vi "Control Panel (New).vi"(8 "error in (no error)":errorcluster, 11 "Lockin SR830 in":refnum<class "Lockin SR830.lvclass">) -> (0 "error out":errorcluster, 3 "Lockin SR830 out":refnum<class "Lockin SR830.lvclass">)   [LabVIEW 2017, in "Lockin SR830.lvclass"]
uses:
  Lockin SR830.lvclass
  Lockin SR830.lvclass/Lockin SR830.ctl
  sr830/SR830.lvlib
panel:
  in  "Read":bool
  in  "Read Dwell Time":dbl[unit] format="%^#_6g"
  out "Ref Freq":dbl[unit]
  out "R":dbl
  out "Y":dbl
  out "X":dbl
  out "Phase":dbl format="%#_13g"
  in  "autophase":bool
  out "External ref":bool=TRUE
  in  "External ref?":bool=TRUE
  in  "Read settings":bool
  in  "Copy actual to set":bool
  in  "Populate fields with member data":bool
  in  "endprgm":bool
  in  "set":bool
  out "sensdisp":T1(ring) caption="Sensitivity"
  out "tcdisp":T2(ring) caption="Time Const."
  in  "sens":T1(ring) caption="Sensitivity"
  in  "tc":T2(ring) caption="Time Const."
  # "Lock-in Detector Front Panel"
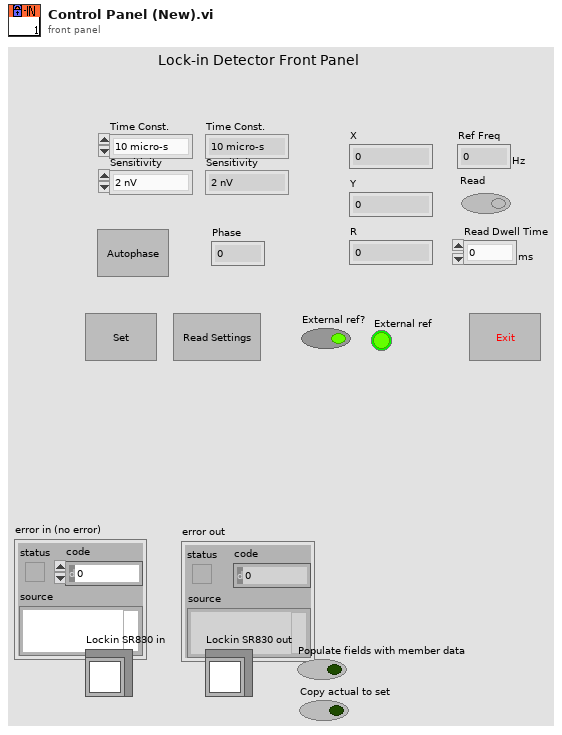
[diagram p1: front panel]
types:
  T1 = enum16{"2 nV", "5 nV", "10 nV", "20 nV", "50 nV", "100 nV", "200 nV", "500 nV", "1 microV", "2 microV", "5 microV", "10 microV", "20 microV", "50  microV", "100  microV", "200  microV", "500  microV", "1 mV", "2 mV", "5 mV", "10 mV", "20 mV", "50 mV", "100 mV", "200  mV", "500 mV", "1 V"}
  T2 = enum16{"10 micro-s", "30 micro-s", "100 micro-s", "300 micro-s", "1 ms", "3 ms", "10 ms", "30 ms", "100 ms", "300 ms", "1 s", "3 s", "10 s", "30 s", "100 s", "300 s", "1000 s", "30000 s", "10 ks", "30 ks"}
  T3 = typedef "Lockin SR830.lvclass/Sensitivity.ctl" = u16
  T4 = typedef "SR830.lvlib/Tau.ctl" = u16
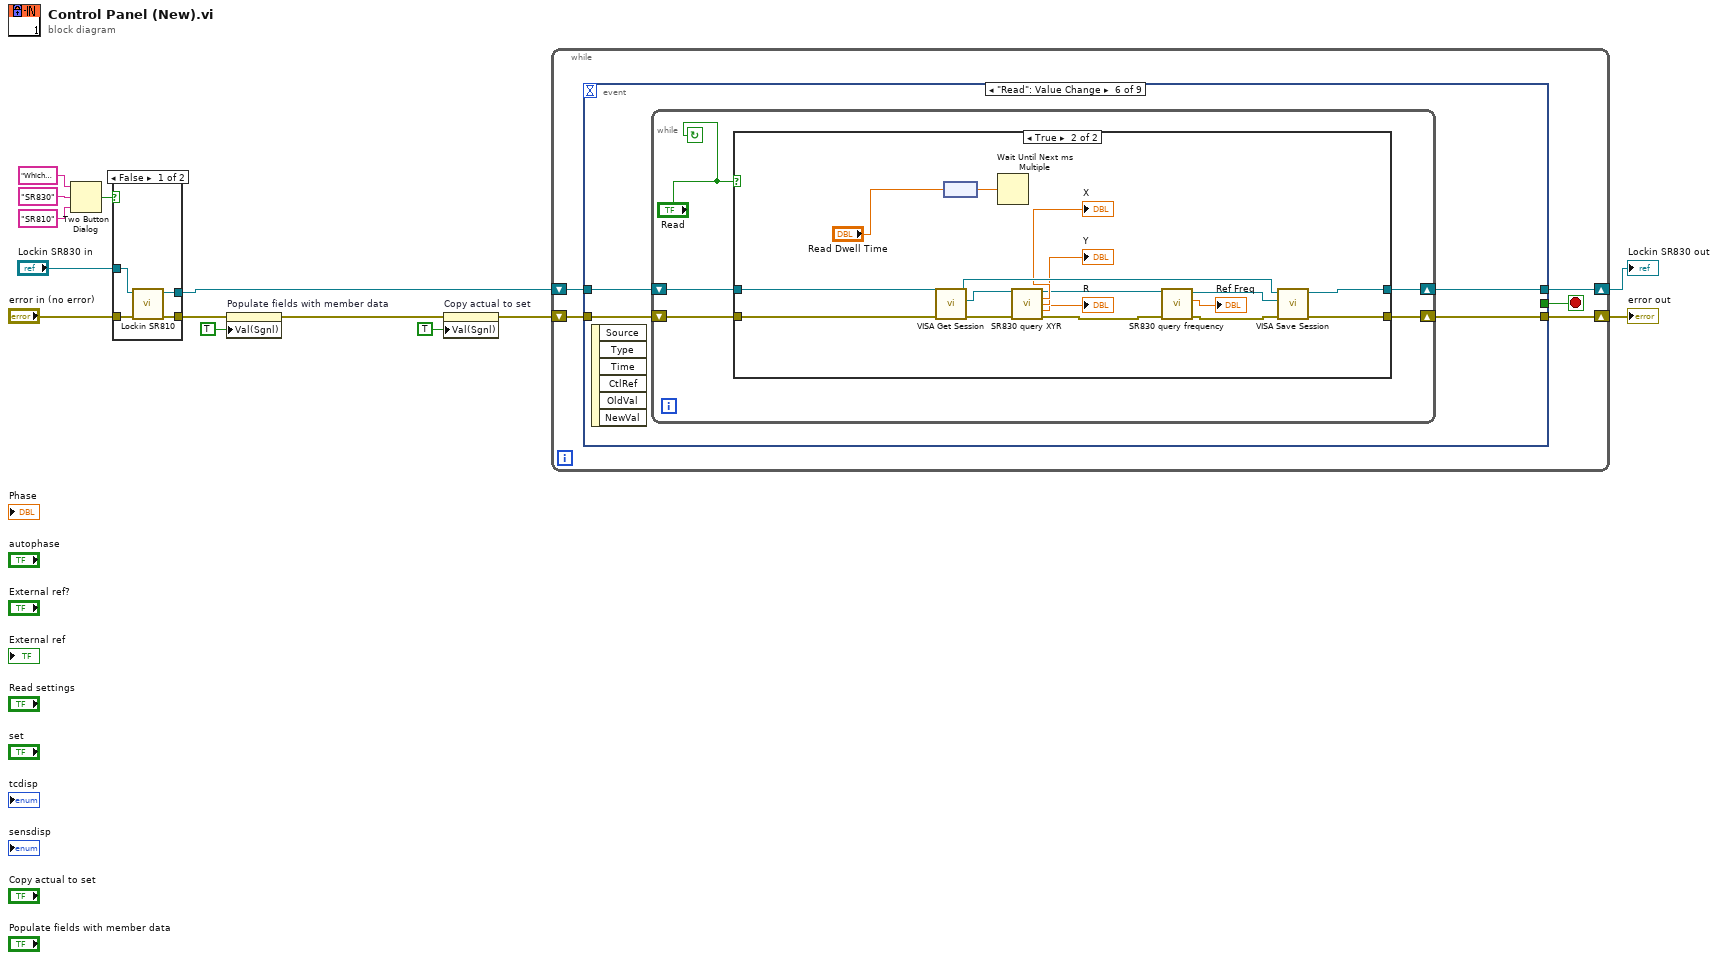
[diagram p0: block diagram]
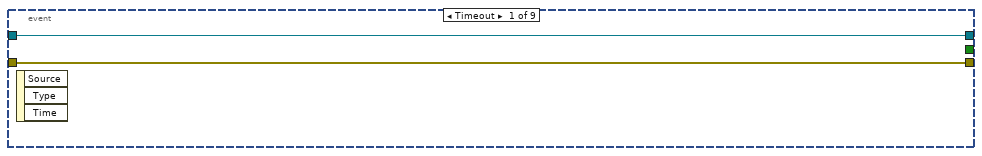
[diagram p2: hidden frame]
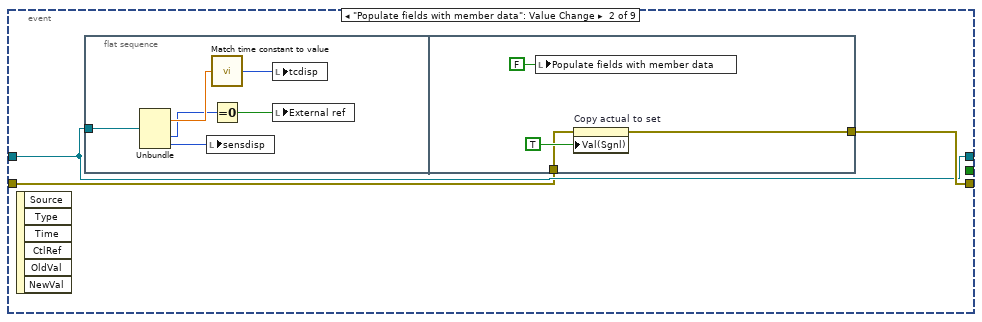
[diagram p3: hidden frame]
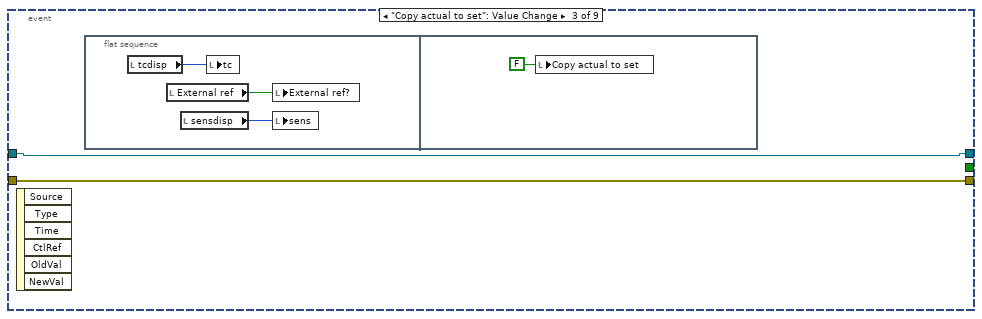
[diagram p4: hidden frame]
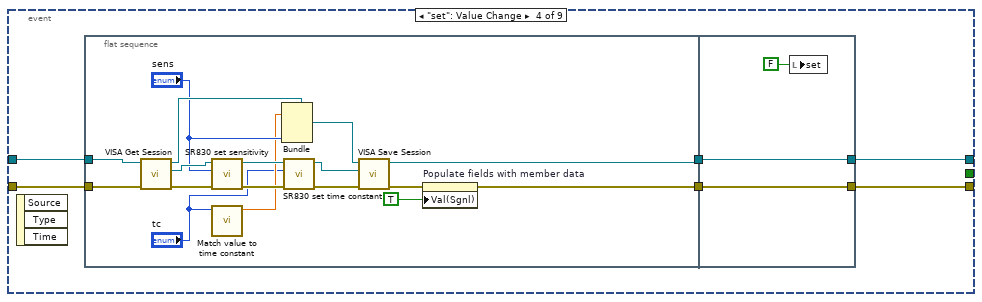
[diagram p5: hidden frame]
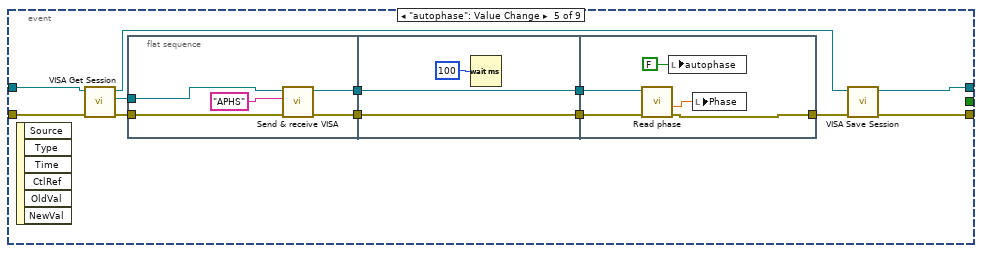
[diagram p6: hidden frame]
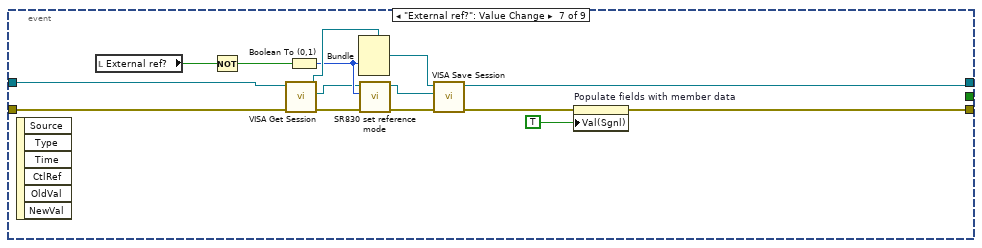
[diagram p8: hidden frame]
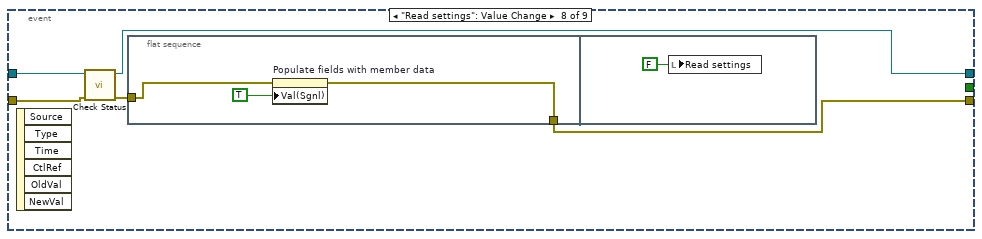
[diagram p9: hidden frame]
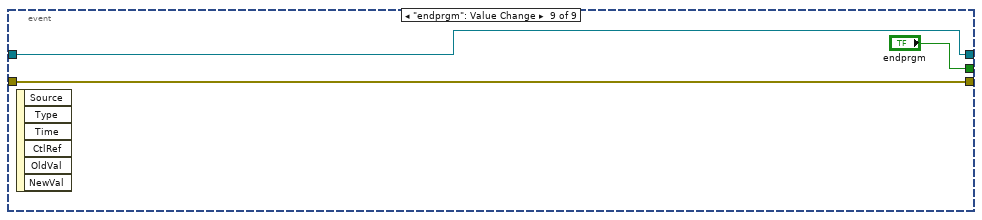
[diagram p10: hidden frame]
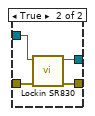
[diagram p11: hidden frame]
diagram:
  n1 = Two Button Dialog(message="Which model Lock-In are you using?", 1:"SR810" ("F button name (\"Cancel\")"), 2:"SR830" ("T button name (\"OK\")")) -> (T button?=w3:bool)
  n2 = case shown="False" w3 {
    tunnel: "Lockin SR830 in" -> [w18 w22]
    tunnel: "error in (no error)" -> [w16 w21]
    tunnel: [w15 w20] -> w7
    tunnel: [w17 w19] -> w1
    frame False {
      n3 = call "Lockin SR810.vi"("error in (no error)"=w16, "Lockin SR830 in"=w18) -> ("error out"=w15:errorcluster, "Lockin SR830 out"=w17:refnum<class "Lockin SR830.lvclass">)  [unwired: 8 in]
    }
    frame True {
      n4 = call "Lockin SR830.vi"("error in (no error)"=w21, "Lockin SR830 in"=w22) -> ("error out"=w20:errorcluster, "Lockin SR830 out"=w19:refnum<class "Lockin SR830.lvclass">)  [unwired: 8 in]
    }
  }
  n5 = property on="Populate fields with member data" class="Bool (strict)"(error in=w7, "Val(Sgnl)"=TRUE) -> (error out=w6:errorcluster)  [unwired: 1 in, 1 out]
  n6 = property on="Copy actual to set" class="Bool (strict)"(error in=w6, "Val(Sgnl)"=TRUE) -> (error out=w2:errorcluster)  [unwired: 1 in, 1 out]
  n7 = while {
    shift-right: [w25] -> w12
    shift-left: w1 -> [w23]
    shift-right: [w26] -> w8
    shift-left: w2 -> [w24]
    stop <- w27 stop-if-true
    n8 = event shown="[5] \"Read\": Value Change" {
      selector: _ -> [_ _ _ _ _ _ _ _ _]
      dyn-events: _ -> [_ _ _ _ _ _ _ _ _]
      timeout: _ -> [_ _ _ _ _ _ _ _ _]
      tunnel: [_ _ _ _ _ _ _ _ "endprgm"] -> w27
      tunnel: [w28 w32 w43 w54 w77 w101 w132 w146 w152] -> w26
      tunnel: [w29 w31 w44 w53 w85 w100 w133 w145 w153] -> w25
      tunnel: w23 -> [w29 w31 w44 w50 w76 w103 w128 w144 w153]
      tunnel: w24 -> [w28 w30 w43 w49 w75 w102 w129 w143 w152]
      event Timeout {
        n9 = event-data() -> ()  [unwired: 1 in, 3 out]
      }
      event "Populate fields with member data": Value Change {
        n10 = event-data() -> ()  [unwired: 1 in, 6 out]
        n11 = flat-sequence {
          tunnel: w31 -> [w37]
          tunnel: [w39] -> w32
          tunnel: w30 -> [w40]
          frame #0 {
            n12 = Unbundle(w37) -> (w36:dbl[unit], w33:enum16{"external", "internal"}, w38:T3)  [unwired: 2 out]
            n13 = local write "sensdisp"(w38) -> ()
            n14 = call "Match time constant to value.vi"("Time constant"=w36) -> ("Tau"=w35:T4)
            n15 = Equal To 0?(x=w33) -> (x = 0?=w34:bool)
            n16 = local write "tcdisp"(w35) -> ()
            n17 = local write "External ref"(w34) -> ()
          }
          frame #1 {
            n18 = local write "Populate fields with member data"(FALSE) -> ()
            n19 = property on="Copy actual to set" class="Bool (strict)"(error in=w40, "Val(Sgnl)"=TRUE) -> (error out=w39:errorcluster)  [unwired: 1 in, 1 out]
          }
        }
      }
      event "Copy actual to set": Value Change {
        n20 = event-data() -> ()  [unwired: 1 in, 6 out]
        n21 = flat-sequence {
          frame #0 {
            n22 = local read "tcdisp"() -> (w47:T2)
            n23 = local read "External ref"() -> (w45:bool)
            n24 = local read "sensdisp"() -> (w46:T1)
            n25 = local write "tc"(w47) -> ()
            n26 = local write "External ref?"(w45) -> ()
            n27 = local write "sens"(w46) -> ()
          }
          frame #1 {
            n28 = local write "Copy actual to set"(FALSE) -> ()
          }
        }
      }
      event "set": Value Change {
        n29 = event-data() -> ()  [unwired: 1 in, 3 out]
        n30 = flat-sequence {
          tunnel: w50 -> [w71]
          tunnel: w49 -> [w69]
          tunnel: [w62] -> w52
          tunnel: [w65] -> w51
          tunnel: [w73] -> w53
          tunnel: [w74] -> w54
          tunnel: w52 -> [w74]
          tunnel: w51 -> [w73]
          frame #0 {
            n31 = call-dynamic "VISA Get Session.vi"("error in (no error)"=w69, "Instrument.lvclass in"=w71) -> ("error out"=w68:errorcluster, "VISA Resource Name"=w70:refnum<visa-resource-name>, "Instrument.lvclass out"=w61:refnum<class "Lockin SR830.lvclass">)  [unwired: 7 out]
            n32 = call "SR830 set sensitivity.vi"("error in (no error)"=w68, "Sensitivity"="sens", "VISA resource name"=w70) -> ("error out"=w66:errorcluster, "VISA resource name out"=w67:refnum<visa-resource-name>)  [unwired: 7 in]
            n33 = call "Match value to time constant.vi"("Tau"="tc") -> ("time constant"=w58:dbl[unit])  [unwired: 10 in]
            n34 = Bundle(cluster=w61, w58, "sens") -> (w59:refnum<class "Lockin SR830.lvclass">)  [unwired: 3 in]
            n35 = call "SR830 set time constant.vi"("error in (no error)"=w66, "Tau"="tc", "VISA resource name"=w67) -> ("error out"=w56:errorcluster, "VISA resource name out"=w55:refnum<visa-resource-name>)  [unwired: 7 in]
            n36 = call-dynamic "VISA Save Session.vi"("error in (no error)"=w56, "VISA Resource Name"=w55, "Instrument.lvclass in"=w59) -> ("error out"=w63:errorcluster, "Instrument.lvclass out"=w65:refnum<class "Lockin SR830.lvclass">)  [unwired: 7 out]
            n37 = property on="Populate fields with member data" class="Bool (strict)"(error in=w63, "Val(Sgnl)"=TRUE) -> (error out=w62:errorcluster)  [unwired: 1 in, 1 out]
          }
          frame #1 {
            n38 = local write "set"(FALSE) -> ()
          }
        }
      }
      event "autophase": Value Change {
        n39 = event-data() -> ()  [unwired: 1 in, 6 out]
        n40 = call-dynamic "VISA Get Session.vi"("error in (no error)"=w75, "Instrument.lvclass in"=w76) -> ("error out"=w83:errorcluster, "VISA Resource Name"=w84:refnum<visa-resource-name>, "Instrument.lvclass out"=w86:refnum<class "Lockin SR830.lvclass">)  [unwired: 7 out]
        n41 = flat-sequence {
          tunnel: w84 -> [w91]
          tunnel: w83 -> [w90]
          tunnel: [w88] -> w81
          tunnel: [w87] -> w79
          tunnel: [w93] -> w82
          tunnel: w81 -> [w93]
          tunnel: [w92] -> w80
          tunnel: w79 -> [w92]
          tunnel: w82 -> [w99]
          tunnel: w80 -> [w98]
          tunnel: [w96] -> w78
          frame #0 {
            n42 = call "Send & receive VISA.vi"("error in (no error)"=w90, "write buffer"="APHS", "VISA resource name"=w91) -> ("error out"=w87:errorcluster, "VISA resource name out"=w88:refnum<visa-resource-name>)  [unwired: 5 in, 2 out]
          }
          frame #1 {
            n43 = Wait (ms)(milliseconds to wait=u32 100) -> ()  [unwired: 1 out]
          }
          frame #2 {
            n44 = call "Read phase.vi"("error in (no error)"=w98, "VISA resource name"=w99) -> ("error out"=w96:errorcluster, "phase"=w97:dbl)  [unwired: 7 in, 1 out]
            n45 = local write "autophase"(FALSE) -> ()
            n46 = local write "Phase"(w97) -> ()
          }
        }
        n47 = call-dynamic "VISA Save Session.vi"("error in (no error)"=w78, "Instrument.lvclass in"=w86) -> ("error out"=w77:errorcluster, "Instrument.lvclass out"=w85:refnum<class "Lockin SR830.lvclass">)  [unwired: 1 in, 7 out]
      }
      event "Read": Value Change {
        n48 = event-data() -> ()  [unwired: 1 in, 6 out]
        n49 = while {
          shift-right: [w105] -> w100
          shift-left: w103 -> [w108]
          shift-right: [w106] -> w101
          shift-left: w102 -> [w107]
          stop <- "Read" continue-if-true
          n50 = case shown="True" "Read" {
            tunnel: w108 -> [w110 w127]
            tunnel: w107 -> [w109 w126]
            tunnel: [w110 w125] -> w105
            tunnel: [w109 w124] -> w106
            frame False {
            }
            frame True {
              n51 = call-dynamic "VISA Get Session.vi"("error in (no error)"=w126, "Instrument.lvclass in"=w127) -> ("error out"=w121:errorcluster, "VISA Resource Name"=w122:refnum<visa-resource-name>, "Instrument.lvclass out"=w123:refnum<class "Lockin SR830.lvclass">)  [unwired: 7 out]
              n52 = node("Read Dwell Time") -> (w112:dbl)
              n53 = Wait Until Next ms Multiple(millisecond multiple=w112) -> ()  [unwired: 1 out]
              n54 = call "SR830 query XYR.vi"("VISA resource name"=w122, "error in (no error)"=w121) -> ("VISA resource name out"=w117:refnum<visa-resource-name>, "X"=→"X":dbl, "Y"=→"Y":dbl, "R"=→"R":dbl, "error out"=w116:errorcluster)  [unwired: 9 in]
              n55 = call "SR830 query frequency.vi"("error in (no error)"=w116, "VISA resource name"=w117) -> ("error out"=w114:errorcluster, "frequency"=→"Ref Freq":dbl[unit], "VISA resource name out"=w115:refnum<visa-resource-name>)  [unwired: 7 in]
              n56 = call-dynamic "VISA Save Session.vi"("error in (no error)"=w114, "VISA Resource Name"=w115, "Instrument.lvclass in"=w123) -> ("error out"=w124:errorcluster, "Instrument.lvclass out"=w125:refnum<class "Lockin SR830.lvclass">)  [unwired: 7 out]
            }
          }
        }
      }
      event "External ref?": Value Change {
        n57 = event-data() -> ()  [unwired: 1 in, 6 out]
        n58 = local read "External ref?"() -> (w135:bool)
        n59 = Not(x=w135) -> (.not. x?=w136:bool)
        n60 = call-dynamic "VISA Get Session.vi"("error in (no error)"=w129, "Instrument.lvclass in"=w128) -> ("error out"=w131:errorcluster, "VISA Resource Name"=w130:refnum<visa-resource-name>, "Instrument.lvclass out"=w140:refnum<class "Lockin SR830.lvclass">)  [unwired: 7 out]
        n61 = Boolean To (0,1)(Boolean=w136) -> (0, 1=w134:i16)
        n62 = Bundle(cluster=w140, w134) -> (w139:refnum<class "Lockin SR830.lvclass">)  [unwired: 4 in]
        n63 = call "SR830 set reference mode.vi"("error in (no error)"=w131, "reference mode"=w134, "VISA resource name"=w130) -> ("error out"=w138:errorcluster, "VISA resource name out"=w137:refnum<visa-resource-name>)  [unwired: 7 in]
        n64 = call-dynamic "VISA Save Session.vi"("error in (no error)"=w138, "VISA Resource Name"=w137, "Instrument.lvclass in"=w139) -> ("error out"=w141:errorcluster, "Instrument.lvclass out"=w133:refnum<class "Lockin SR830.lvclass">)  [unwired: 7 out]
        n65 = property on="Populate fields with member data" class="Bool (strict)"(error in=w141, "Val(Sgnl)"=TRUE) -> (error out=w132:errorcluster)  [unwired: 1 in, 1 out]
      }
      event "Read settings": Value Change {
        n66 = event-data() -> ()  [unwired: 1 in, 6 out]
        n67 = call-dynamic "Check Status.vi"("error in (no error)"=w143, "Lockin SR830 in"=w144) -> ("error out"=w147:errorcluster, "Lockin SR830 out"=w145:refnum<class "Lockin SR830.lvclass">)  [unwired: 6 in, 2 out]
        n68 = flat-sequence {
          tunnel: w147 -> [w149]
          tunnel: [w148] -> w146
          frame #0 {
            n69 = property on="Populate fields with member data" class="Bool (strict)"(error in=w149, "Val(Sgnl)"=TRUE) -> (error out=w148:errorcluster)  [unwired: 1 in, 1 out]
          }
          frame #1 {
            n70 = local write "Read settings"(FALSE) -> ()
          }
        }
      }
      event "endprgm": Value Change {
        n71 = event-data() -> ()  [unwired: 1 in, 6 out]
      }
    }
  }
  "error out" <- w8
  "Lockin SR830 out" <- w12
